vi "subVI verify RSSI saved_demoinfocom.vi"(8 "Configuration:Active Antenna":string, 9 "Configuration:Carrier Frequency":dbl, 10 "error in (no error)":errorcluster, 11 "reference":refnum<k15>) -> (2 "error out":errorcluster, 3 "reference out":refnum<k15>)   [LabVIEW 2021]
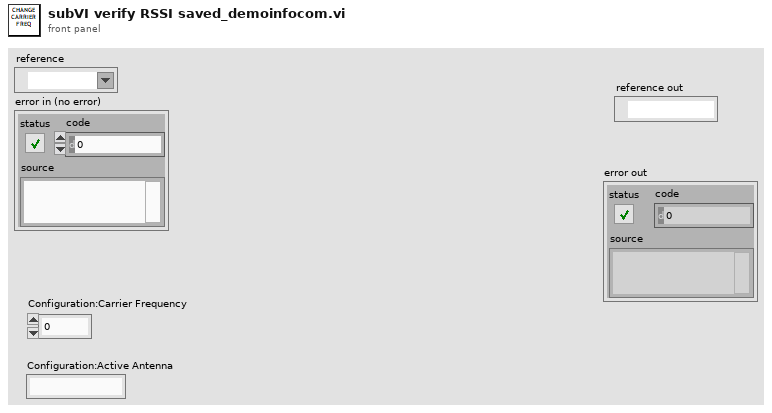
[diagram p1: front panel]
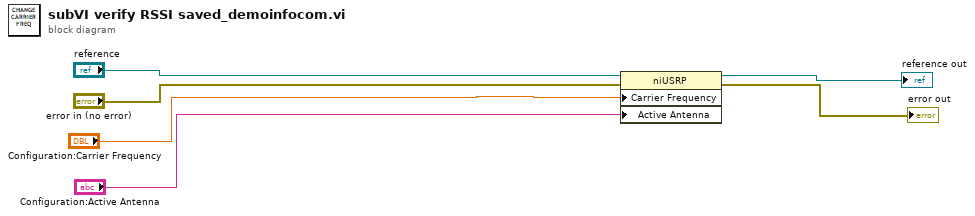
[diagram p0: block diagram]
diagram:
  n1 = property class="niUSRP"(reference="reference", error in="error in (no error)", "Carrier Frequency"="Configuration:Carrier Frequency", "Active Antenna"="Configuration:Active Antenna") -> (reference out=→"reference out":refnum<k15>, error out=→"error out":errorcluster)
